vi "convert.vi"(8 "error in (no error)":errorcluster, 10 "inputs":dbl[](array[numeric]), 11 "TTLConverter in":refnum<class "TTLConverter.lvclass">) -> (0 "error out":errorcluster, 2 "outputs":u8[](array[numeric]), 3 "TTLConverter out":refnum<class "TTLConverter.lvclass">)   [LabVIEW 2017, in "TTLConverter.lvclass"]
doc: "Convert an array of dbl to an array of uint8, which can be feed into digital write vi (as port)"
uses:
  TTLConverter.lvclass
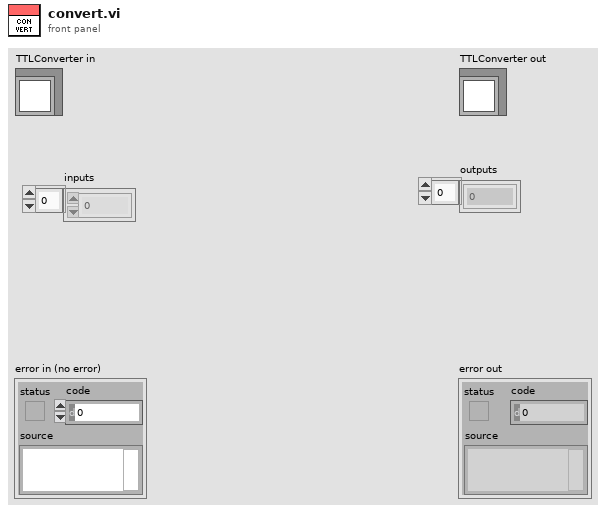
[diagram p1: front panel]
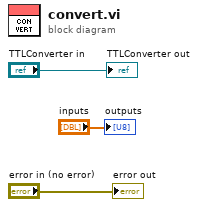
[diagram p0: block diagram]
diagram:
  "error out" <- "error in (no error)"
  "TTLConverter out" <- "TTLConverter in"
  "outputs" <- "inputs"
